vi "Ping.vi"(8 "Error In":errorcluster, 11 "CS++RTMainActor in":refnum<class "CS++RTMainActor.lvclass">) -> (0 "Error Out":errorcluster, 3 "CS++RTMainActor out":refnum<class "CS++RTMainActor.lvclass">)   [LabVIEW 2016, in "CS++RTMain.lvlib" / "CS++RTMainActor.lvclass"]
doc: "Increment Ping Counter and publish to SV."
uses:
  CS++RTMainActor.lvclass
  CS++RTMainActor.lvclass/CS++RTMainActor.ctl
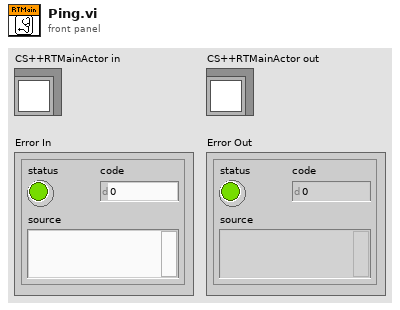
[diagram p1: front panel]
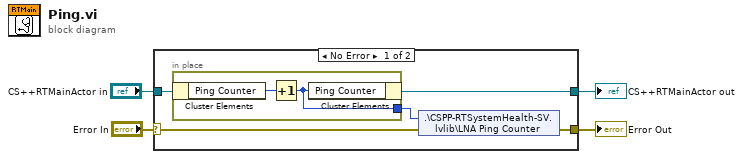
[diagram p0: block diagram]
diagram:
  n1 = case shown="No Error" "Error In" {
    selector: "Error In" -> [w6 w13]
    tunnel: [w5 w13] -> w1
    tunnel: [w8 w12] -> w3
    tunnel: "CS++RTMainActor in" -> [w9 w12]
    frame No Error {
      n2 = in-place {
        in-place-border: [w10] -> w7
        n3 = in-place-cluster #1(w9) -> ("Ping Counter"=w11:u64)
        n4 = Increment(x=w11) -> (x+1=w10:u64)
        n5 = in-place-cluster #1("Ping Counter"=w10) -> (w8:refnum<class "CS++RTMainActor.lvclass">)
      }
      n6 = shared-variable ".\\CSPP-RTSystemHealth-SV.lvlib\\LNA Ping Counter"(w7, error in=w6) -> (error out=w5:errorcluster)
    }
    frame Error {
    }
  }
  "Error Out" <- w1
  "CS++RTMainActor out" <- w3
